vi "Prepare Tree Entries.vi"(11 "Entries":cluster{"Entry IDs":T1[], "Names":string[]}) -> (2 "Tokens":string[](array[string]), 3 "Sorted Tree Rows":cluster{"Array":string[], "Field ID":T1}[](array[cluster]))   [LabVIEW 2017]
uses:
  <vilib>/Rock Robotics/Network Tables/Field ID.ctl
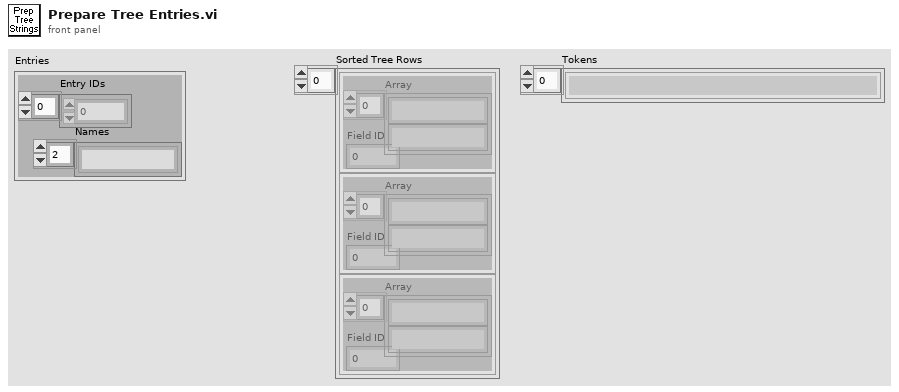
[diagram p1: front panel]
types:
  T1 = typedef "Field ID.ctl" = i32
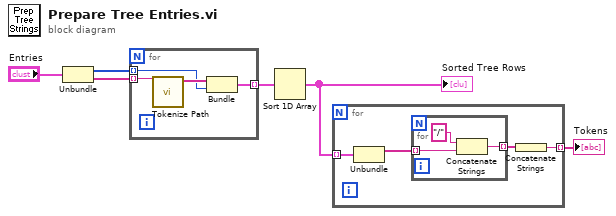
[diagram p0: block diagram]
diagram:
  n1 = Unbundle("Entries") -> ("Entry IDs"=w4:T1[], "Names"=w5:string[])
  n2 = for {
    tunnel: w5 -> [w10] mode=indexing
    tunnel: w4 -> [w8] mode=indexing
    tunnel: [w7] -> w3 mode=indexing
    n3 = call <vilib>:"Tokenize Path.vi"("Name"=w10) -> ("Array"=w9:string[])  [unwired: 10 in]
    n4 = Bundle("Array"=w9, "Field ID"=w8) -> (w7:cluster{"Array":string[], "Field ID":T1})  [unwired: 1 in]
  }
  n5 = Sort 1D Array(array=w3) -> (sorted array=w2:cluster{"Array":string[], "Field ID":T1}[])
  "Sorted Tree Rows" <- w2
  n6 = for {
    tunnel: w2 -> [w14] mode=indexing
    tunnel: [w11] -> w1 mode=indexing
    n7 = Unbundle(w14) -> ("Array"=w13:string[])  [unwired: 1 out]
    n8 = for {
      tunnel: w13 -> [w16] mode=indexing
      tunnel: [w15] -> w12 mode=indexing
      n9 = Concatenate Strings("/", w16) -> (w15:string)
    }
    n10 = Concatenate Strings(w12) -> (w11:string)
  }
  "Tokens" <- w1
